vi "actuate_singleManipJumpExp_v0.03.vi"(0 "Phase Cluster":T3, 1 "valve Time Cluster":T2, 3 "data in":T4={"daq_ao 1"="Dev1/ao0", "daq_ai 1"="Dev1/ai0", "experiment day folder"=path "D:/DATA/8-27-15 save func testing/test.lvm", "Multiclamp init error"=0, "Multiclamp Handle Out"=0, "sampling rate (Hz)"=10000, "trial name"=""}, 5 "PhaseLetter":string, 7 "controls array in":refnum<vi>[](array[refnum]), 9 "time to wait for solution change (min)":dbl=2.5 min=0.0 step=0.01, 11 "error in":errorcluster, 12 "common cluster":T6, 13 "individual controls in":T5) -> (4 "output cluster":T1={"daq_ao 2"="", "Duration (s)"=0.0, "Sample Freq (Hz)"=0.0, "Phase"=0.0, "Duty Cycle"=0.0, "Jump Filter Freq (Hz)"=0.0, "Number of Replicates"=1} {"Number of Replicates" min=1 max=10}, 6 "protocol waveform":waveform(dbl)(graph), 8 "protcol response":waveform(dbl)[](graph) caption="protocol response", 10 "control array out":refnum<vi>[](array[refnum]), 14 "experiment VI ref":refnum<vi>, 15 "error out":errorcluster)   [LabVIEW 2019]
uses:
  controls/scope_motion.ctl
  pipette cleaning/pressure box/cleaning_soft/controls/actuator_type.ctl
  pipette cleaning/pressure box/cleaning_soft/controls/actuator_cluster.ctl
  machine_vision/coordinate model vis/transform_properties_actuators.ctl
  machine_vision/controls/transform_cluster_actuator.ctl
  controls/NH_method.ctl
  pipette cleaning/pressure box/cleaning_soft/controls/pressure_box_type.ctl
  pipette cleaning/pressure box/cleaning_soft/controls/pressure_box_control.ctl
  multipatch/controls/multipatch_common_controls_v4.ctl
  controls/memtest_def.ctl
  multipatch/controls/multipatch_individual_controls_v5.ctl
  Controls/Data.ctl
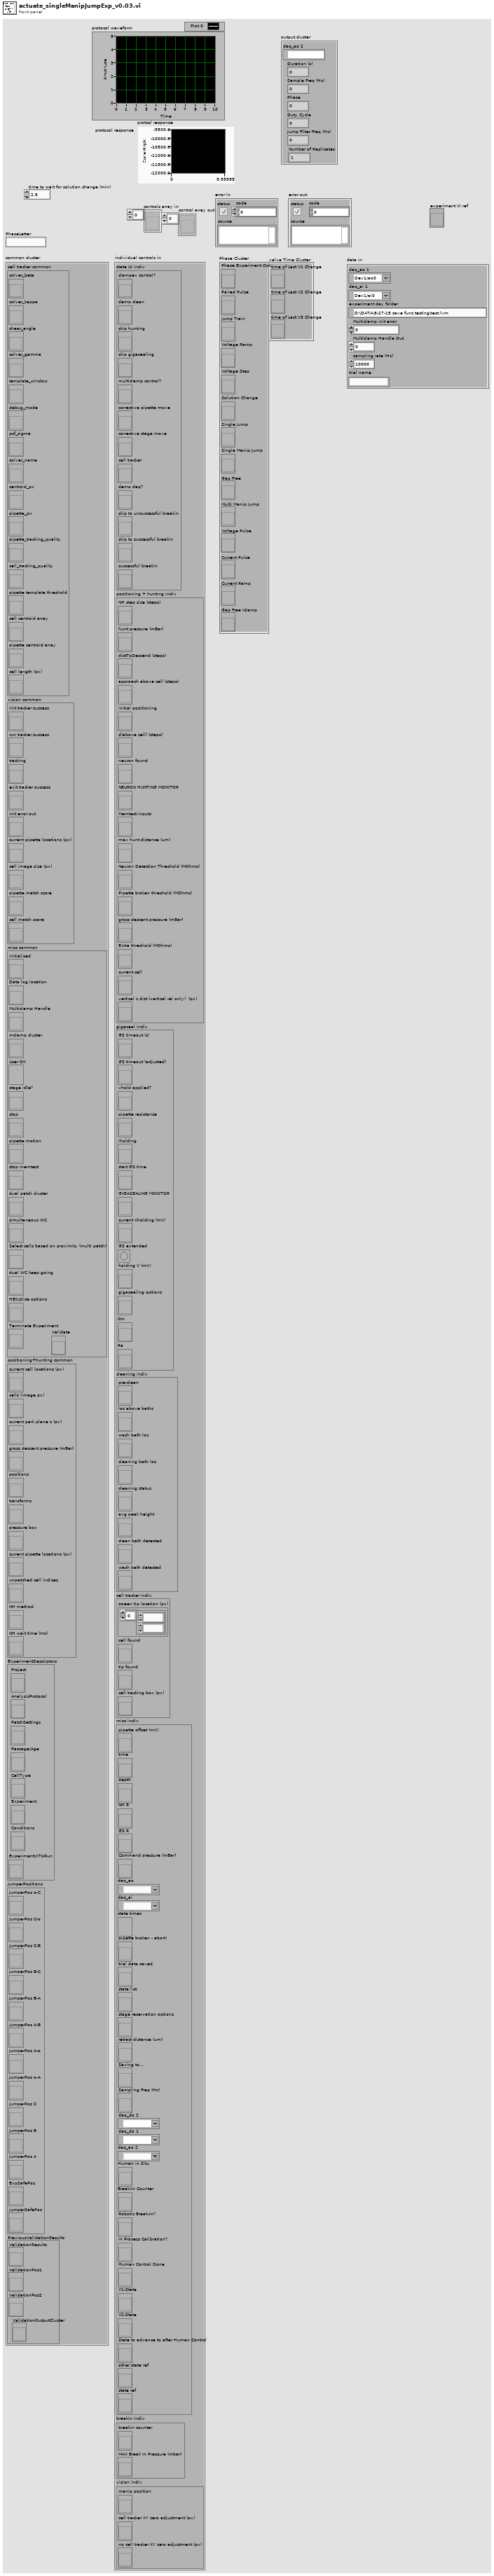
[diagram p1: front panel]
types:
  T1 = cluster{"daq_ao 2":tag, "Duration (s)":dbl, "Sample Freq (Hz)":dbl, "Phase":dbl, "Duty Cycle":dbl, "Jump Filter Freq (Hz)":dbl, "Number of Replicates":i16}
  T2 = cluster{"time of Last V1 Change":refnum<vi>, "time of Last V2 Change":refnum<vi>, "time of Last V3 Change":refnum<vi>}
  T3 = cluster{"Phase Experiment Option":refnum<vi>, "Paired Pulse":refnum<vi>, "Jump Train":refnum<vi>, "Voltage Ramp":refnum<vi>, "Voltage Step":refnum<vi>, "Solution Change":refnum<vi>, "Single Jump":refnum<vi>, "Single Manip Jump":refnum<vi>, "Gap Free":refnum<vi>, "Multi Manip Jump":refnum<vi>, "Voltage Pulse":refnum<vi>, "Current Pulse":refnum<vi>, "Current Ramp":refnum<vi>, "Gap Free Iclamp":refnum<vi>}
  T4 = typedef "Data.ctl" = cluster{"daq_ao 1":tag, "daq_ai 1":tag, "experiment day folder":path, "Multiclamp init error":i32, "Multiclamp Handle Out":u32, "sampling rate (Hz)":i32, "trial name":string}
  T5 = typedef "multipatch_individual_controls_v5.ctl" = cluster{"state UI indiv":cluster{"clampex control?":refnum<vi>, "demo clean":refnum<vi>, "skip hunting":refnum<vi>, "skip gigasealing":refnum<vi>, "multiclamp control?":refnum<vi>, "corrective pipette move":refnum<vi>, "corrective stage move":refnum<vi>, "cell tracker":refnum<vi>, "demo daq?":refnum<vi>, "skip to unsuccessful breakin":refnum<vi>, "skip to successful breakin":refnum<vi>, "successful breakin":refnum<vi>}, "positioning + hunting indiv":cluster{"NH step size (steps)":refnum<vi>, "hunt pressure (mBar)":refnum<vi>, "distToDescend (steps)":refnum<vi>, "approach above cell (steps)":refnum<vi>, "initial positioning":refnum<vi>, "d(above cell) (steps)":refnum<vi>, "neuron found":refnum<vi>, "NEURON HUNTING MONITOR":refnum<vi>, "Memtest inputs":refnum<vi>, "max hunt distance (um)":refnum<vi>, "Neuron Detection Threshold (MOhms)":refnum<vi>, "Pipette broken threshold (MOhms)":refnum<vi>, "gross descent pressure (mBar)":refnum<vi>, "Extra threshold (MOhms)":refnum<vi>, "current cell":refnum<vi>, "vertical z dist (vertical rel only)  (px)":refnum<vi>}, "gigaseal indiv":cluster{"GS timeout (s)":refnum<vi>, "GS timeout (adjusted)":refnum<vi>, "vhold applied?":refnum<vi>, "pipette resistance":refnum<vi>, "Iholding":refnum<vi>, "start GS time":refnum<vi>, "GIGASEALING MONITOR":refnum<vi>, "current Vholding (mV)":refnum<vi>, "GS extended":refnum<vi>, "holding V (mV)":refnum<vi>, "gigasealing options":refnum<vi>, "Cm":refnum<vi>, "Ra ":refnum<vi>}, "cleaning indiv":cluster{"pre-clean":refnum<vi>, "loc above baths":refnum<vi>, "wash bath loc":refnum<vi>, "cleaning bath loc":refnum<vi>, "cleaning status":refnum<vi>, "avg peak height":refnum<vi>, "clean bath detected":refnum<vi>, "wash bath detected":refnum<vi>}, "cell tracker indiv":cluster{"screen tip location (px)":refnum<vi>, "cell found":refnum<vi>, "tip found":refnum<vi>, "cell tracking box (px)":refnum<vi>}, "misc indiv":cluster{"pipette offset (mV)":refnum<vi>, "time":refnum<vi>, "depth":refnum<vi>, "NH R":refnum<vi>, "GS R":refnum<vi>, "Command pressure (mBar)":refnum<vi>, "daq_ao":tag, "daq_ai":tag, "state times":refnum<vi>, "pipette broken - abort!":refnum<vi>, "trial data saved":refnum<vi>, "state list":refnum<vi>, "stage reservation options":refnum<vi>, "retract distance (um)":refnum<vi>, "Saving to...":refnum<vi>, "Sampling Freq (Hz)":refnum<vi>, "daq_do 2":tag, "daq_do 1":tag, "daq_ao 2":tag, "Human in Situ":refnum<vi>, "Break-In Counter":refnum<vi>, "Robotic Break-In?":refnum<vi>, "In Process Calibration?":refnum<vi>, "Human Control Done":refnum<vi>, "V1-State":refnum<vi>, "V2-State":refnum<vi>, "State to advance to after Human Control":refnum<vi>, "other state ref":refnum<vi>, "state ref":refnum<vi>}, "breakin indiv":cluster{"breakin counter":refnum<vi>, "MAX Break In Pressure (mbar)":refnum<vi>}, "vision indiv":cluster{"manip position":refnum<vi>, "cell tracker XY zero adjustment (px)":refnum<vi>, "no cell tracker XY zero adjustment (px)":refnum<vi>}}
  T6 = typedef "multipatch_common_controls_v4.ctl" = cluster{"cell tracker common":cluster{"solver_beta":refnum<vi>, "solver_kappa":refnum<vi>, "shear_angle":refnum<vi>, "solver_gamma":refnum<vi>, "template_window":refnum<vi>, "debug_mode":refnum<vi>, "psf_sigma":refnum<vi>, "solver_name":refnum<vi>, "centroid_px":refnum<vi>, "pipette_px":refnum<vi>, "pipette_tracking_quality":refnum<vi>, "cell_tracking_quality":refnum<vi>, "pipette template threshold":refnum<vi>, "cell centroid array":refnum<vi>, "pipette centroid array":refnum<vi>, "cell length (px)":refnum<vi>}, "vision common":cluster{"init tracker success":refnum<vi>, "run tracker success":refnum<vi>, "tracking":refnum<vi>, "exit tracker success":refnum<vi>, "init error out":refnum<vi>, "current pipette locations (px)":refnum<vi>, "cell image size (px)":refnum<vi>, "pipette match score":refnum<vi>, "cell match score":refnum<vi>}, "misc common":cluster{"initialized":refnum<vi>, "Data log location":refnum<vi>, "Multiclamp Handle":refnum<vi>, "mclamp cluster":refnum<vi>, "User OK":refnum<vi>, "stage idle?":refnum<vi>, "stop":refnum<vi>, "pipette motion":refnum<vi>, "stop memtest":refnum<vi>, "dual patch cluster":refnum<vi>, "simultaneous WC":refnum<vi>, "Select cells based on proximity (multi patch)":refnum<vi>, "dual WC keep going":refnum<vi>, "HEK/slice options":refnum<vi>, "Terminate Experiment":refnum<vi>, "Validate":refnum<vi>}, "positioning+hunting common":cluster{"current cell locations (px)":refnum<vi>, "cells (image px)":refnum<vi>, "current park plane z (px)":refnum<vi>, "gross descent pressure (mBar)":refnum<vi>, "positions":refnum<vi>, "transforms":refnum<vi>, "pressure box":refnum<vi>, "current pipette locations (px)":refnum<vi>, "unpatched cell indices":refnum<vi>, "NH method":refnum<vi>, "NH wait time (ms)":refnum<vi>}, "ExperimentDescriptors":cluster{"Project":refnum<vi>, "AnalysisProtocol":refnum<vi>, "PatchSettings":refnum<vi>, "Passage/Age":refnum<vi>, "CellType":refnum<vi>, "Experiment":refnum<vi>, "Conditions":refnum<vi>, "ExperimentVIToRun":refnum<vi>}, "JumperPositions":cluster{"JumperPos o-C":refnum<vi>, "JumperPos C-o":refnum<vi>, "JumperPos C-B":refnum<vi>, "JumperPos B-C":refnum<vi>, "JumperPos B-A":refnum<vi>, "JumperPos A-B":refnum<vi>, "JumperPos A-o":refnum<vi>, "JumperPos o-A":refnum<vi>, "JumperPos C":refnum<vi>, "JumperPos B":refnum<vi>, "JumperPos A":refnum<vi>, "ExpSafePos":refnum<vi>, "jumperSafePos":refnum<vi>}, "PreviousValidationResults":cluster{"ValidationResults":refnum<vi>, "ValidationPos1":refnum<vi>, "ValidationPos2":refnum<vi>, "ValidationOutputCluster":refnum<vi>}}
  T7 = cluster{"Start Position (N)":enum16{"Jumper Safe Position", "Experiment Safe Position", "Jumper Position A", "Jumper Position B", "Jumper Position C", "Jumper Position o-A", "Jumper Position A-o", "Jumper Position A-B", "Jumper Position B-A", "Jumper Position B-C", "Jumper Position C-B", "Jumper Position C-o", "Jumper Position o-C", "Don't Move"}, "Duration (s)":dbl, "Delay (s)":dbl, "Pulse Width (s)":dbl, "Valve 1 Position":i16, "Valve 2 Position":i16, "Replicates":dbl, "Jump Position (m)":enum16{"Jumper Safe Position", "Experiment Safe Position", "Jumper Position A", "Jumper Position B", "Jumper Position C", "Jumper Position o-A", "Jumper Position A-o", "Jumper Position A-B", "Jumper Position B-A", "Jumper Position B-C", "Jumper Position C-B", "Jumper Position C-o", "Jumper Position o-C", "Don't Move"}, "Vholding (mV)":dbl, "Valve 3 Position":i16, "valve 1 used now?":bool, "valve 2 used now?":bool, "valve 3 used now? ":bool, "protocol Preview":waveform(dbl)[]}
  T8 = enum16{"Jumper Safe Position", "Experiment Safe Position", "Jumper Position A", "Jumper Position B", "Jumper Position C", "Jumper Position o-A", "Jumper Position A-o", "Jumper Position A-B", "Jumper Position B-A", "Jumper Position B-C", "Jumper Position C-B", "Jumper Position C-o", "Jumper Position o-C", "Don't Move"}
  T9 = typedef "transform_cluster_actuator.ctl" = cluster{"s":refnum<vi>, "manip 1":refnum<vi>, "manip 2":refnum<vi>, "manip 3":refnum<vi>, "manip 4":refnum<vi>}
  T10 = enum16{"manipulator 1", "manipulator 2", "manipulator 3", "manipulator 4"}
  T11 = typedef "scope_motion.ctl" = enum16{"superSlow", "fast", "slow", "find slice speed", "slow_dualPatch"}
  T12 = typedef "transform_properties_actuators.ctl" = cluster{"theta (deg)":dbl, "X sc factor (px/step)":dbl, "Y sc factor (px/step)":dbl, "zero loc (x,y,z)":dbl[], "flip y?":bool, "flip x?":bool, "gamma (deg)":dbl, "flip z?":bool, "Z sc factor (px/step)":dbl, "actuator":T13, "safe space (steps)":i32[]}
  T13 = typedef "actuator_cluster.ctl" = cluster{"Actuator COM":refnum<visa-resource-name>, "Actuator type":T14}
  T14 = typedef "actuator_type.ctl" = enum16{"Scientifica", "Sutter", "Demo", "Off"}
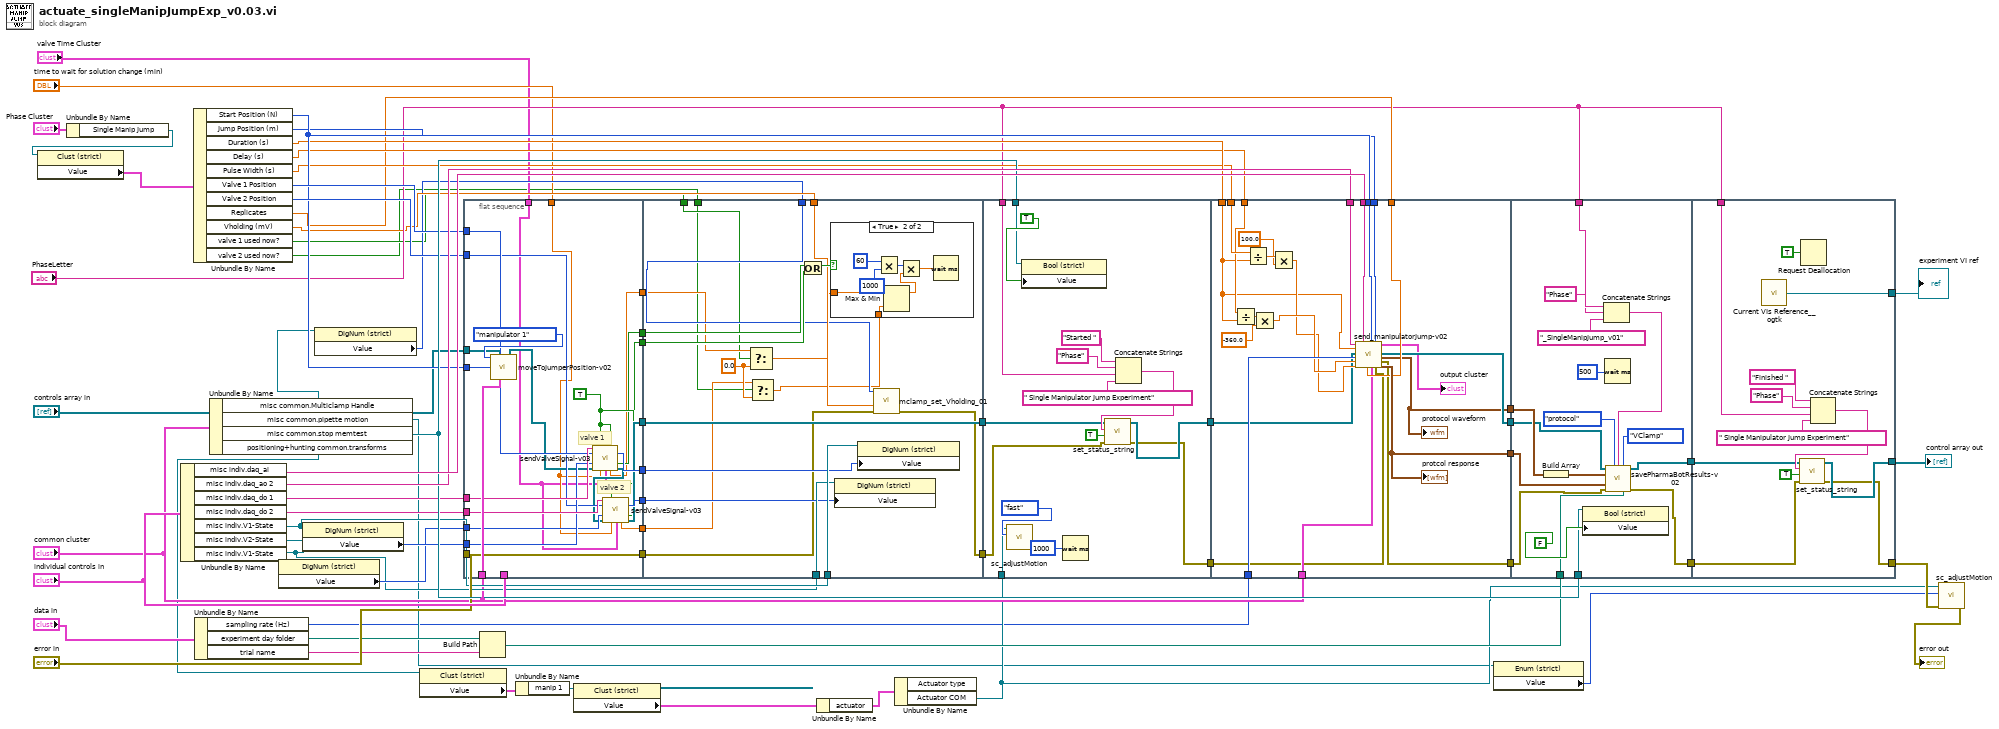
[diagram p0: block diagram]
diagram:
  n1 = Unbundle By Name("Phase Cluster") -> ("Single Manip Jump"=w33:refnum<vi>)
  n2 = property class="Clust (strict)"(reference=w33) -> ("Value"=w32:T7)  [unwired: 1 in, 2 out]
  n3 = Unbundle By Name("individual controls in") -> ("misc indiv.daq_ai"=w67:tag, "misc indiv.daq_ao 2"=w66:tag, "misc indiv.daq_do 1"=w63:tag, "misc indiv.daq_do 2"=w62:tag, "misc indiv.V1-State"=w54:refnum<vi>, "misc indiv.V2-State"=w53:refnum<vi>)  [unwired: 1 out]
  n4 = Unbundle By Name(w32) -> ("Start Position (N)"=w28:T8, "Jump Position (m)"=w27:T8, "Duration (s)"=w26:dbl, "Delay (s)"=w24:dbl, "Pulse Width (s)"=w25:dbl, "Valve 1 Position"=w30:i16, "Valve 2 Position"=w29:i16, "Replicates"=w22:dbl, "Vholding (mV)"=w10:dbl, "valve 1 used now?"=w3:bool, "valve 2 used now?"=w2:bool)
  n5 = Unbundle By Name("data in") -> ("sampling rate (Hz)"=w23:i32, "experiment day folder"=w47:path, "trial name"=w46:string)
  n6 = Unbundle By Name("common cluster") -> ("misc common.Multiclamp Handle"=w9:refnum<vi>, "misc common.pipette motion"=w34:refnum<vi>, "misc common.stop memtest"=w65:refnum<vi>, "positioning+hunting common.transforms"=w41:refnum<vi>)
  n7 = property class="DigNum (strict)"(reference=w53) -> ("Value"=w55:u16)  [unwired: 1 in, 2 out]
  n8 = property class="DigNum (strict)"(reference=w54) -> ("Value"=w56:u16)  [unwired: 1 in, 2 out]
  n9 = property class="DigNum (strict)"(reference=w9) -> ("Value"=w8:u32)  [unwired: 1 in, 2 out]
  n10 = property class="Clust (strict)"(reference=w41) -> ("Value"=w42:T9)  [unwired: 1 in, 2 out]
  n11 = flat-sequence {
    tunnel: "common cluster" -> [w90]
    tunnel: "individual controls in" -> [_]
    tunnel: w63 -> [w89]
    tunnel: w62 -> [w88]
    tunnel: "error in" -> [w87]
    tunnel: [w87] -> w57
    tunnel: w56 -> [w86]
    tunnel: w55 -> [w85]
    tunnel: [w84] -> w52
    tunnel: [w83] -> w51
    tunnel: w28 -> [w81]
    tunnel: w30 -> [w80]
    tunnel: w29 -> [w79]
    tunnel: "controls array in" -> [w78]
    tunnel: [w75] -> w17
    tunnel: [w73] -> w12
    tunnel: [w72] -> w11
    tunnel: "time to wait for solution change (min)" -> [w71]
    tunnel: "valve Time Cluster" -> [w70]
    tunnel: [w69] -> w5
    tunnel: [w68] -> w4
    tunnel: [w99] -> w58
    tunnel: w57 -> [w101]
    tunnel: w54 -> [w109]
    tunnel: w53 -> [w108]
    tunnel: w52 -> [w107]
    tunnel: w51 -> [w106]
    tunnel: [w105] -> w18
    tunnel: w17 -> [w105]
    tunnel: w12 -> [w104]
    tunnel: w11 -> [w102]
    tunnel: w10 -> [w100]
    tunnel: w8 -> [w98]
    tunnel: w5 -> [w96]
    tunnel: w4 -> [w93]
    tunnel: w3 -> [w92]
    tunnel: w2 -> [w91]
    tunnel: w65 -> [w129]
    tunnel: [w118] -> w59
    tunnel: w58 -> [w119]
    tunnel: w36 -> [w127]
    tunnel: [w120] -> w19
    tunnel: w18 -> [w121]
    tunnel: "PhaseLetter" -> [w117]
    tunnel: w67 -> [w154]
    tunnel: w66 -> [w153]
    tunnel: [w136] -> w60
    tunnel: w59 -> [w137]
    tunnel: [w133] -> w50
    tunnel: [w152] -> w49
    tunnel: "common cluster" -> [w138]
    tunnel: w28 -> [w151]
    tunnel: w27 -> [w150]
    tunnel: w26 -> [w140]
    tunnel: w25 -> [w145]
    tunnel: w24 -> [w144]
    tunnel: w23 -> [w143]
    tunnel: w22 -> [w139]
    tunnel: [w134] -> w20
    tunnel: w19 -> [w135]
    tunnel: w65 -> [w170]
    tunnel: w60 -> [w159]
    tunnel: w50 -> [w169]
    tunnel: w49 -> [w167]
    tunnel: w45 -> [w164]
    tunnel: "PhaseLetter" -> [w160]
    tunnel: w20 -> [w158]
    tunnel: [w156] -> w15
    tunnel: [w157] -> w14
    tunnel: [w177] -> w16
    tunnel: [w174] -> w38
    tunnel: w15 -> [w175]
    tunnel: w14 -> [w178]
    tunnel: "PhaseLetter" -> [w176]
    tunnel: [w173] -> w1
    frame #0 {
      w74 = TRUE ("Set Status")
      # "valve 2"
      # "valve 1"
      n12 = call "moveToJumperPosition-v02.vi"("which manipulator"=T10."manipulator 1", "controls array in"=w78, "Which Jumper Position to move to?"=w81, "common cluster"=w90) -> ("control array out"=w77:refnum<vi>[])  [unwired: 10 in, 1 out]
      n13 = call "sendValveSignal-v03.vi"("daq_do"=w89, "Set Status"=w74, "Valve1?"=w74, "ChangeToValve"=w80, "CurrentValve"=w86, "controls array in"=w77, "time to wait for solution change (min)"=w71, "valve Time Cluster"=w70) -> ("ValveSetTo"=w83:u16, "valve changed?"=w73:bool, "additional time to wait (min)"=w69:dbl, "control array out"=w76:refnum<vi>[])  [unwired: 4 in]
      n14 = call "sendValveSignal-v03.vi"("daq_do"=w88, "Set Status"=w74, "ChangeToValve"=w79, "CurrentValve"=w85, "controls array in"=w76, "time to wait for solution change (min)"=w71, "valve Time Cluster"=w70) -> ("ValveSetTo"=w84:u16, "valve changed?"=w72:bool, "additional time to wait (min)"=w68:dbl, "control array out"=w75:refnum<vi>[])  [unwired: 5 in]
    }
    frame #1 {
      w97 = 0.0 ("f")
      n15 = Select(t=w96, s=w92, f=w97) -> (s? t:f=w95:dbl)
      n16 = Select(t=w93, s=w91, f=w97) -> (s? t:f=w94:dbl)
      n17 = Or(x=w104, y=w102) -> (x .or. y?=w103:bool)
      n18 = case shown="True" w103 {
        tunnel: w95 -> [_ w112]
        tunnel: w94 -> [_ w111]
        frame False {
        }
        frame True {
          n19 = Multiply(x=u32 60 ("milliseconds to wait"), y=u32 1000) -> (x*y=w114:u32)
          n20 = Max & Min(x=w112, y=w111) -> (max(x,y)=w110:dbl)  [unwired: 1 out]
          n21 = Multiply(x=w114, y=w110) -> (x*y=w113:dbl)
          n22 = Wait (ms)(milliseconds to wait=w113) -> ()  [unwired: 1 out]
        }
      }
      n23 = property class="DigNum (strict)"(reference=w108, "Value"=w107) -> ()  [unwired: 1 in, 2 out]
      n24 = property class="DigNum (strict)"(reference=w109, "Value"=w106) -> ()  [unwired: 1 in, 2 out]
      n25 = call "mclamp_set_Vholding_01.vi"("error in (no error)"=w101, "set holding (mV)"=w100, "Multiclamp Handle Out"=w98) -> ("error out"=w99:errorcluster)  [unwired: 7 in, 1 out]
    }
    frame #2 {
      n26 = call "sc_adjustMotion.vi"("motion"=scope_motion."fast", "VISA handle"=w127) -> ()  [unwired: 8 in, 2 out]
      n27 = property class="Bool (strict)"(reference=w129, "Value"=TRUE ("stop memtest")) -> ()  [unwired: 1 in, 2 out]
      n28 = Wait (ms)(milliseconds to wait=u32 1000) -> ()  [unwired: 1 out]
      n29 = Concatenate Strings("Started " ("string"), "Phase" ("string"), w117, " Single Manipulator Jump Experiment" ("string")) -> (w123:string)
      n30 = call "set_status_string.vi"("error in"=w119, "new line?"=TRUE, "status string in"=w123, "controls array"=w121) -> ("error out"=w118:errorcluster, "controls array out"=w120:refnum<vi>[])  [unwired: 6 in]
    }
    frame #3 {
      n31 = Divide(x=w144, y=w140) -> (x/y=w146:dbl)
      n32 = Divide(x=w145, y=w140) -> (x/y=w149:dbl)
      n33 = Multiply(x=w146, y=-360.0) -> (x*y=w142:dbl)
      n34 = Multiply(x=w149, y=100.0) -> (x*y=w141:dbl)
      n35 = call "send_manipulatorJump-v02.vi"("daq_ao 2"=w153, "Duration (s)"=w140, "controls array in"=w135, "Sample Freq (Hz)"=w143, "Phase"=w142, "Duty Cycle"=w141, "daq_ai"=w154, "Number of Replicates"=w139, "Start Position"=w151, "common cluster"=w138, "Jump Position"=w150, "error in"=w137) -> ("output cluster"=→"output cluster":T1, "control array out"=w134:refnum<vi>[], "protcol waveform"=w133:waveform(dbl), "error out"=w136:errorcluster, "protcol response"=w152:waveform(dbl)[])  [unwired: 3 in]
      "protcol response" <- w152
      "protocol waveform" <- w133
    }
    frame #4 {
      n36 = Build Array(w169) -> (w168:waveform(dbl)[])
      n37 = property class="Bool (strict)"(reference=w170, "Value"=FALSE ("stop memtest")) -> ()  [unwired: 1 in, 2 out]
      n38 = Concatenate Strings("Phase" ("string"), w160, "_SingleManipJump_v01" ("string")) -> (w161:string)
      n39 = Wait (ms)(milliseconds to wait=u32 500) -> ()  [unwired: 1 out]
      n40 = call "savePharmaBotResults-v02.vi"("controls array"=w158, "protocol or memtest"=enum16{"protocol", "memtest", "validation"}."protocol", "ExpPhase"=w161, "which clamp"=enum16{"VClamp", "IClamp"}."VClamp", "protocol waveform"=w168, "protocol response"=w167, "error in"=w159, "Save to (folder dir)"=w164) -> ("controls array out"=w157:refnum<vi>[], "error out"=w156:errorcluster)  [unwired: 6 in]
    }
    frame #5 {
      n41 = call "Current VIs Reference__ogtk.vi"() -> ("Current VI's reference"=w173:refnum<vi>)  [unwired: 5 in]
      n42 = Request Deallocation(TRUE ("flag")) -> ()
      n43 = Concatenate Strings("Finished " ("string"), "Phase" ("string"), w176, " Single Manipulator Jump Experiment" ("string")) -> (w180:string)
      n44 = call "set_status_string.vi"("error in"=w175, "new line?"=TRUE, "status string in"=w180, "controls array"=w178) -> ("error out"=w174:errorcluster, "controls array out"=w177:refnum<vi>[])  [unwired: 6 in]
    }
  }
  n45 = Build Path(base path=w47, name or relative path=w46) -> (appended path=w45:path)
  n46 = Unbundle By Name(w42) -> ("manip 1"=w43:refnum<vi>)
  n47 = property class="Clust (strict)"(reference=w43) -> ("Value"=w40:T12)  [unwired: 1 in, 2 out]
  n48 = Unbundle By Name(w40) -> ("actuator"=w39:T13)
  n49 = Unbundle By Name(w39) -> ("Actuator COM"=w36:refnum<visa-resource-name>)  [unwired: 1 out]
  n50 = property class="Enum (strict)"(reference=w34) -> ("Value"=w35:T11)  [unwired: 1 in, 2 out]
  n51 = call "sc_adjustMotion.vi"("error in (no error)"=w38, "motion"=w35, "VISA handle"=w36) -> ("error out"=→"error out":errorcluster)  [unwired: 7 in, 1 out]
  "control array out" <- w16
  "experiment VI ref" <- w1
